vi "Sending String Data Only.vi"(0 "TCP Ref In":refnum<k5>, 1 "Time Out(ms)":i32=100, 2 "Re-Try":i32=5, 5 "Data":string, 11 "error in (no error)":errorcluster) -> (4 "TCP Ref Out":refnum<k5>, 15 "error out":errorcluster)   [LabVIEW 2024]
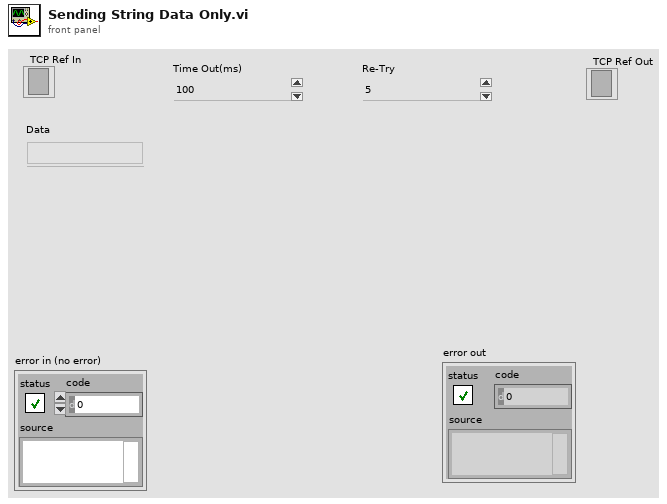
[diagram p1: front panel]
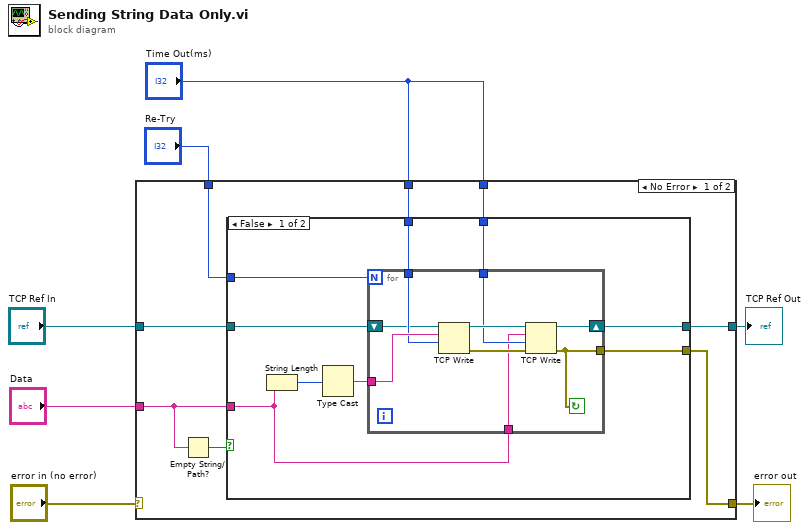
[diagram p0: block diagram]
diagram:
  n1 = case shown="No Error" "error in (no error)" {
    selector: "error in (no error)" -> [_ w36]
    tunnel: [w15 w36] -> w6
    tunnel: "Data" -> [w12 _]
    tunnel: "Time Out(ms)" -> [w14 _]
    tunnel: "Time Out(ms)" -> [w13 _]
    tunnel: "TCP Ref In" -> [w11 w35]
    tunnel: [w9 w35] -> w2
    tunnel: "Re-Try" -> [w8 _]
    frame No Error {
      n2 = Empty String/Path?(string/path=w12) -> (empty?=w10:bool)
      n3 = case shown="False" w10 {
        tunnel: [w23 _] -> w15
        tunnel: w14 -> [w22 _]
        tunnel: w13 -> [w21 _]
        tunnel: [w20 w34] -> w9
        tunnel: w12 -> [w18 _]
        tunnel: w11 -> [w19 w34]
        tunnel: w8 -> [w16 _]
        frame False {
          n4 = String Length(string=w18) -> (length=w17:i32)
          n5 = Type Cast(x=w17) -> (*(type *) &x=w24:string)  [unwired: 1 in]
          n6 = for {
            N: w16 -> [_]
            tunnel: w24 -> [w31]
            tunnel: [w25] -> w23
            tunnel: w22 -> [w30]
            tunnel: w21 -> [w29]
            tunnel: w18 -> [w26]
            shift-right: [w28] -> w20
            shift-left: w19 -> [w27]
            stop <- w25 continue-if-true
            n7 = TCP Write(connection ID=w27, data in=w31, 9:w30) -> (connection ID out=w32:refnum<k5>, error out=w33:errorcluster)  [unwired: 1 in, 1 out]
            n8 = TCP Write(connection ID=w32, data in=w26, error in (no error)=w33, 9:w29) -> (connection ID out=w28:refnum<k5>, error out=w25:errorcluster)  [unwired: 1 out]
          }
        }
        frame True {
        }
      }
    }
    frame Error {
    }
  }
  "error out" <- w6
  "TCP Ref Out" <- w2
